vi "Get Context Dependent Ring.vi"(0 "cds":cluster{"Strings":string[]}[][](array[cluster]), 7 "rings":i32[][](array[numeric]), 11 "Cell Position":T1) -> (4 "Strings":string[](array[string]))   [LabVIEW 2015, in "KTable.xctl"]
uses:
  KTable.xctl
  <vilib>/Utility/miscctls.llb/LVRowAndColumnTypeDef.ctl
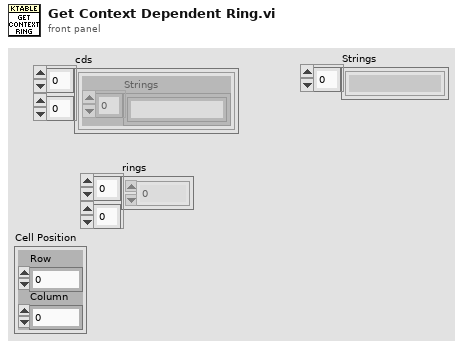
[diagram p1: front panel]
types:
  T1 = typedef "LVRowAndColumnTypeDef.ctl" = cluster{"Row":i32, "Column":i32}
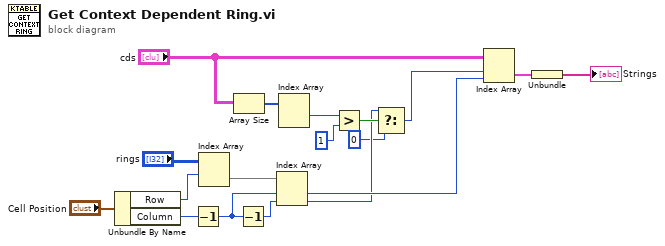
[diagram p0: block diagram]
diagram:
  n1 = Unbundle By Name("Cell Position") -> ("Row"=w16:i32, "Column"=w12:i32)
  n2 = Decrement(x=w12) -> (x-1=w7:i32)
  n3 = Index Array(array="rings", index (row)=w16) -> (element=w13:i32[])  [unwired: 1 in]
  n4 = Array Size(array="cds") -> (size(s)=w14:i32[])
  n5 = Decrement(x=w7) -> (x-1=w6:i32)
  n6 = Index Array(array=w13, index #1=w7, index #2=w6) -> (element #1=w11:i32, element #2=w4:i32)
  n7 = Index Array(array=w14) -> (element #1=w9:i32)  [unwired: 2 in, 1 out]
  n8 = Greater?(x=w9, y=1) -> (0:w5:bool)
  n9 = Select(t=w4, s=w5, f=0) -> (s? t:f=w3:i32)
  n10 = Index Array(array="cds", index (row)=w3, index (col)=w11) -> (element=w10:cluster{"Strings":string[]})
  n11 = Unbundle(w10) -> ("Strings"=→"Strings":string[])
